vi "x-axis.vi"(8 "error in (no error)":errorcluster, 11 "Voltage Pulse Gating System (HV supply) in":refnum<class "Voltage Pulse Gating System (HV supply).lvclass">) -> (0 "error out":errorcluster, 1 "Label":string, 2 "Unit":string, 3 "Voltage Pulse Gating System (HV supply) out":refnum<class "Voltage Pulse Gating System (HV supply).lvclass">)   [LabVIEW 2017, in "Voltage Pulse Gating System (HV supply).lvclass"]
uses:
  Voltage Pulse Gating System (HV supply).lvclass
  Scanner/Scanner.lvclass
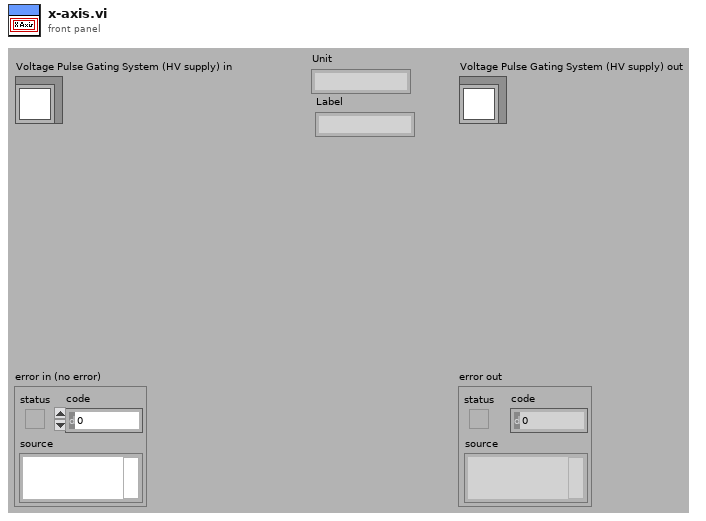
[diagram p1: front panel]
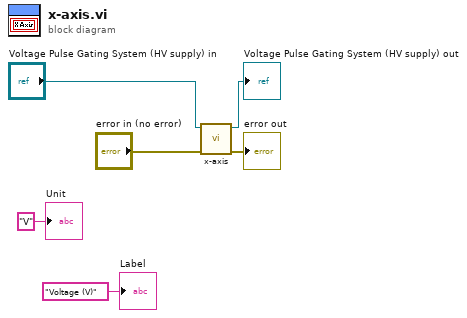
[diagram p0: block diagram]
diagram:
  n1 = call-parent "x-axis.vi"("error in (no error)"="error in (no error)", "Scanner in"="Voltage Pulse Gating System (HV supply) in") -> ("error out"=→"error out":errorcluster, "Scanner out"=→"Voltage Pulse Gating System (HV supply) out":refnum<class "Voltage Pulse Gating System (HV supply).lvclass">)  [unwired: 6 in, 2 out]
  "Label" <- "Voltage (V)" ("Label")
  "Unit" <- "V" ("Unit")
